vi "Lock.vi"(8 "error in (no error)":errorcluster, 10 "Password":string, 11 "Session in":refnum<k21>) -> (0 "error out":errorcluster, 3 "Session out":refnum<k21>)   [LabVIEW 2014, in "nisyscfg.lvlib"]
doc: "Enables a system or device to be locked."
uses:
  nisyscfg.lvlib
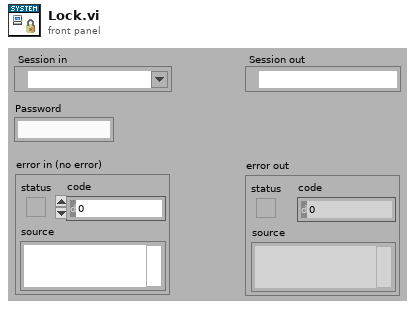
[diagram p1: front panel]
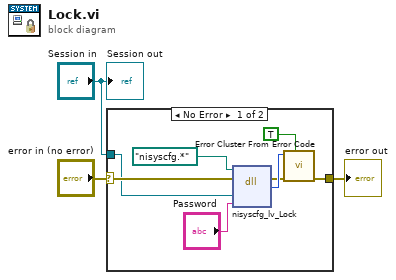
[diagram p0: block diagram]
diagram:
  n1 = case shown="No Error" "error in (no error)" {
    selector: "error in (no error)" -> [w7 w12]
    tunnel: [w10 w12] -> w3
    tunnel: "Session in" -> [w6 _]
    frame No Error {
      n2 = dll-call lib="nisyscfg.*" fn="nisyscfg_lv_Lock" label="Lock"(path in=path "nisyscfg.*", error in=w7, "system"=w6, "password"="Password") -> (error out=w8:errorcluster, "result"=w9:i32)  [unwired: 3 in, 1 out]
      n3 = call "Error Cluster From Error Code.vi"("show call chain? (False)"=TRUE, "error in (no error)"=w8, "error code (0)"=w9) -> ("error out"=w10:errorcluster)  [unwired: 6 in]
    }
    frame Error {
    }
  }
  "error out" <- w3
  "Session out" <- "Session in"
